vi "Pack Control.vi"(7 "s":bool, 10 "Total elements":u32, 11 "Elements wrote in":u32) -> (2 "Elements wrote out":u32, 3 "Output Valid":bool)   [LabVIEW 2015]
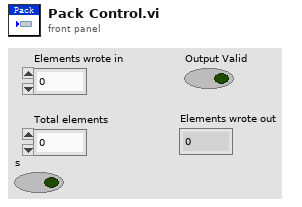
[diagram p1: front panel]
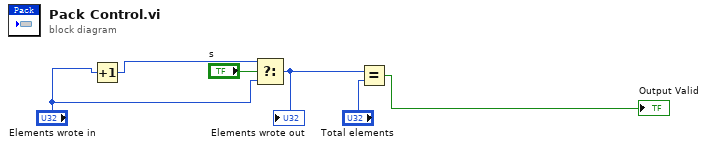
[diagram p0: block diagram]
diagram:
  n1 = Increment(x="Elements wrote in") -> (x+1=w2:u32)
  n2 = Select(t=w2, s="s", f="Elements wrote in") -> (s? t:f=w5:u32)
  "Elements wrote out" <- w5
  n3 = Equal?(x=w5, y="Total elements") -> (x = y?=→"Output Valid":bool)
